vi "Logika case v13.vi"() -> ()   [LabVIEW 2014]
uses:
  Timer/Timer 2013/Control Timer.ctl
panel:
  in  "lokalna B3":bool
  out "Trenutno stanje":T1(ring)
  out "flag":dbl
  out "error out":errorcluster
  in  "error in (no error)":errorcluster
  in  "Stanja":T1(ring)
  in  "Flag":enum16{"1", "2", "3"}(ring)
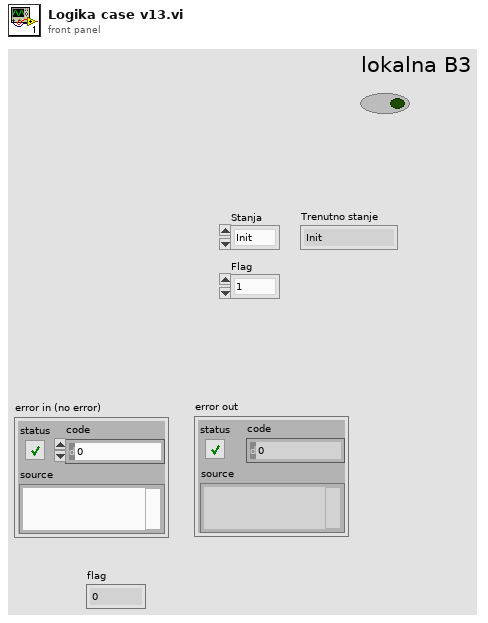
[diagram p1: front panel]
types:
  T1 = enum16{"Init", "Wait", "na1", "na2", "na3", "ispredLifta", "idiNaLift", "naLiftu", "uNivou1", "stigao1", "podizanje", "uNivou2", "stigao2", "uNivou3", "stigao3", "SHUTDOWN", "visak1", "visak2", "visak3"}
  T2 = typedef "Control Timer.ctl" = enum16{"Timecheck", "Reset"}
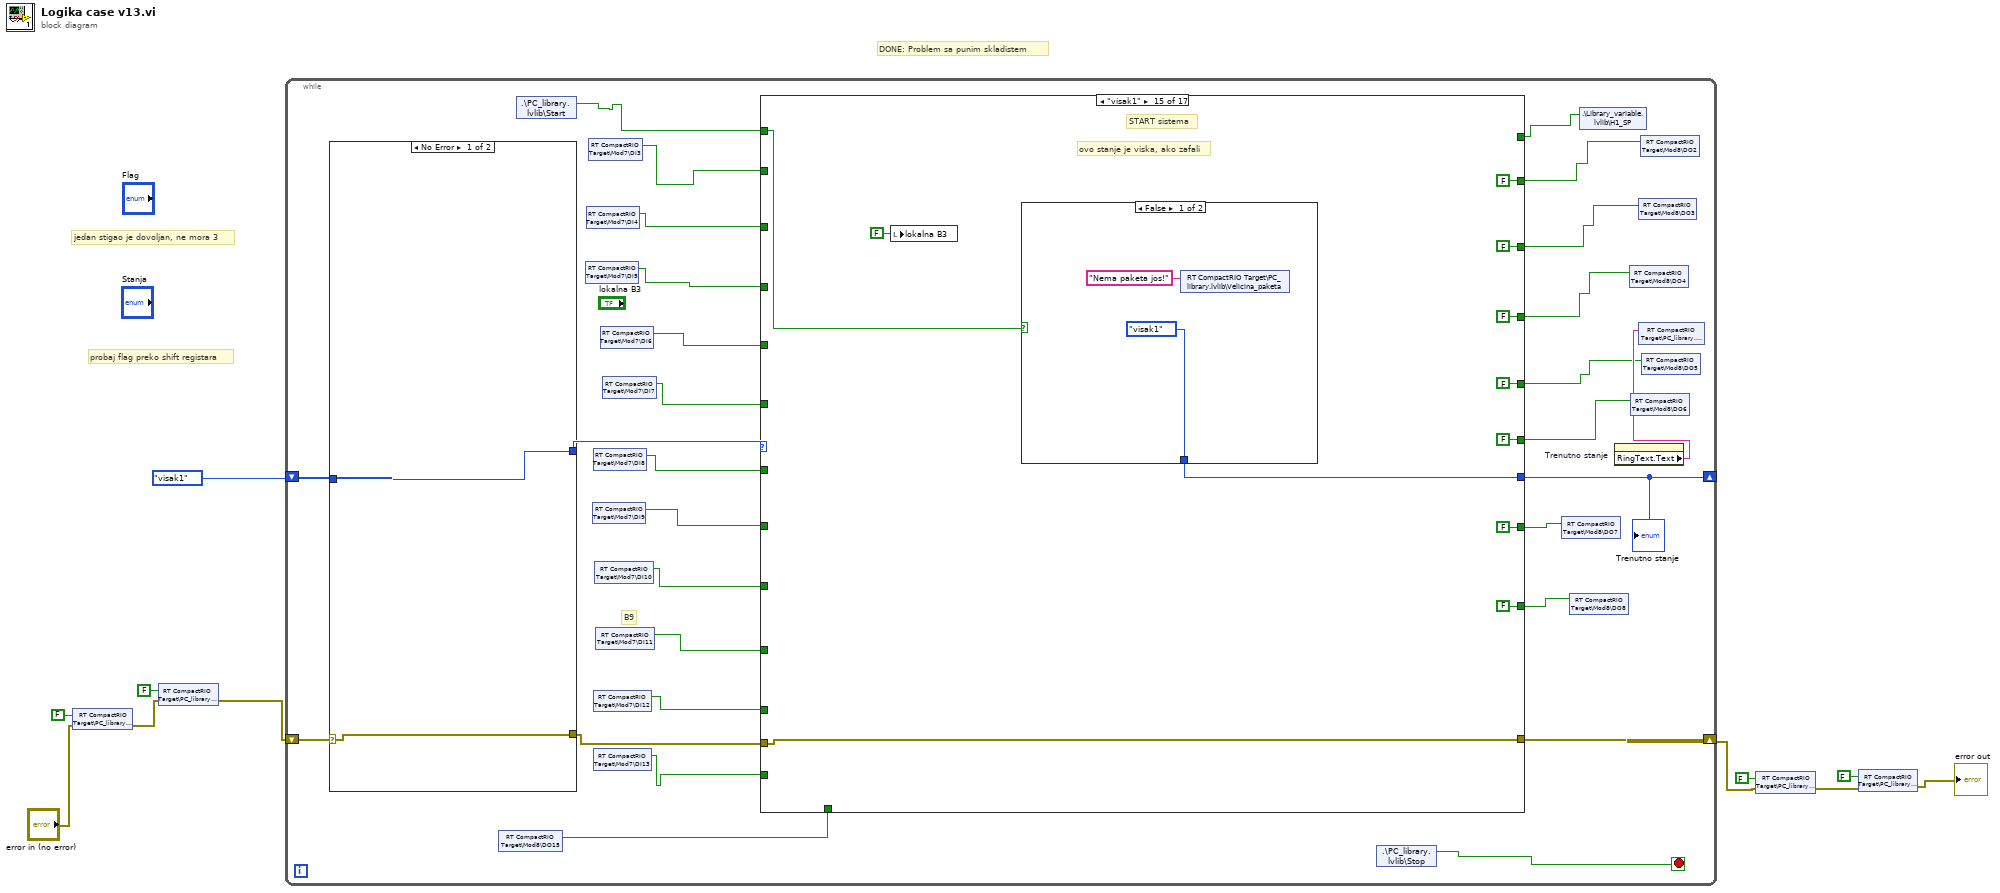
[diagram p0: block diagram]
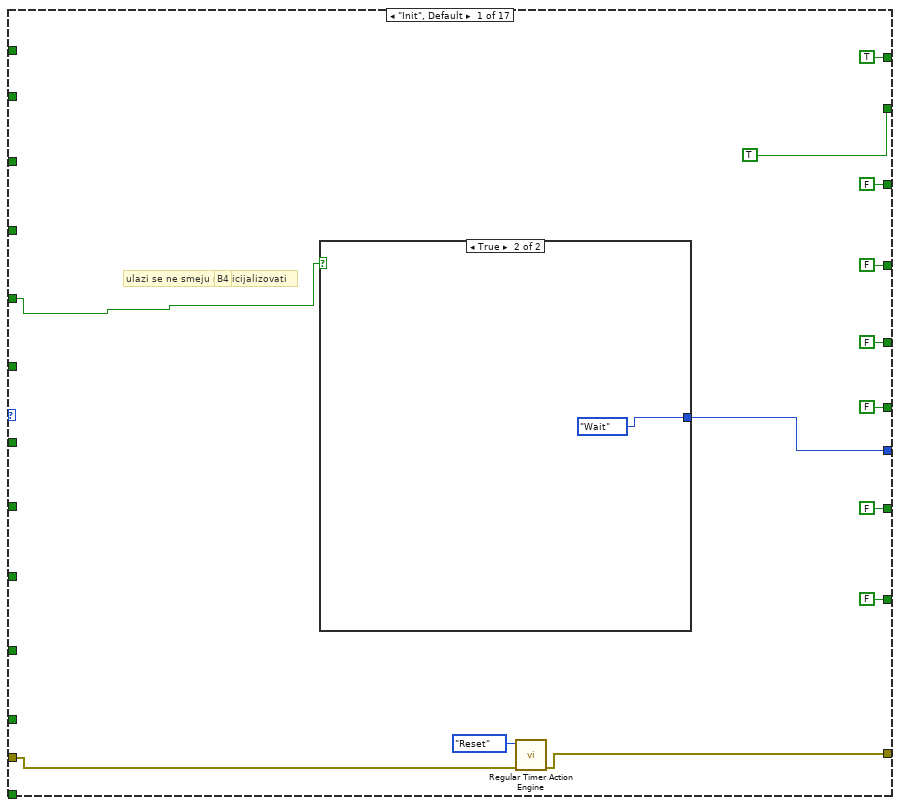
[diagram p2: hidden frame]
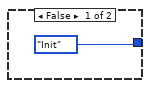
[diagram p3: hidden frame]
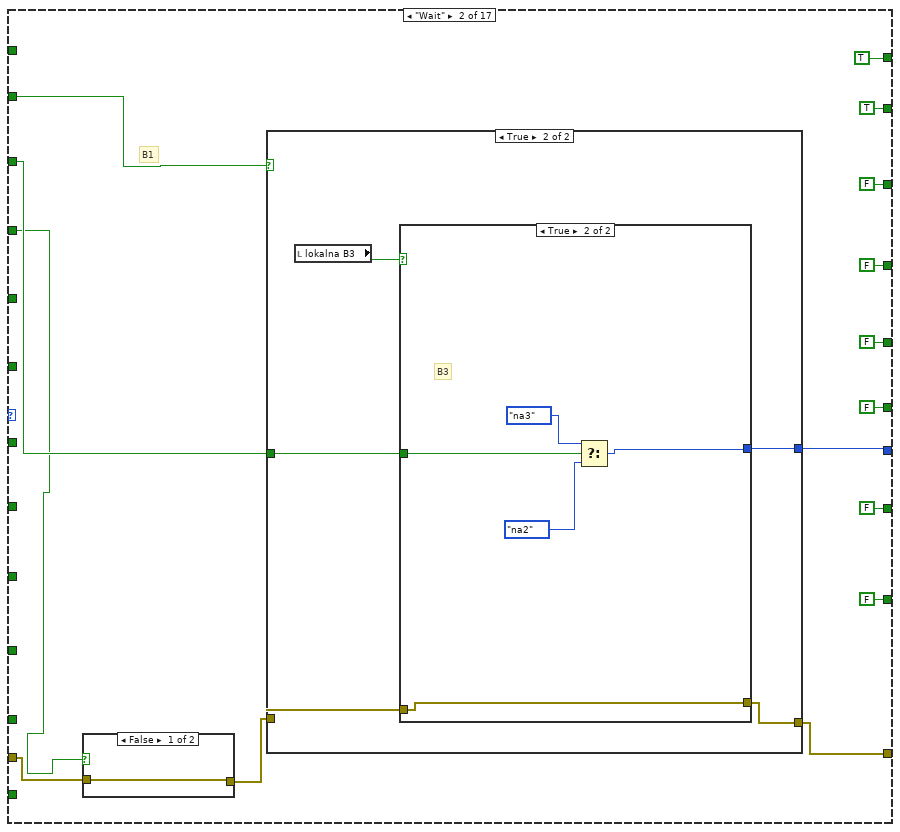
[diagram p4: hidden frame]
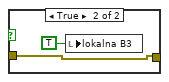
[diagram p5: hidden frame]
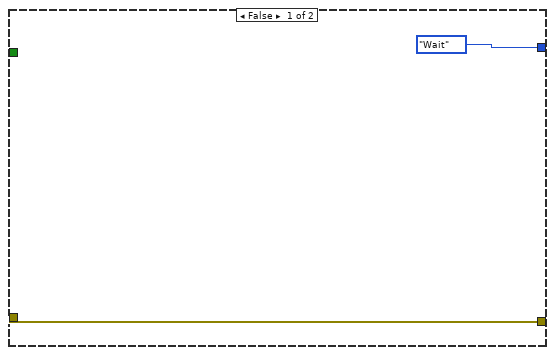
[diagram p6: hidden frame]
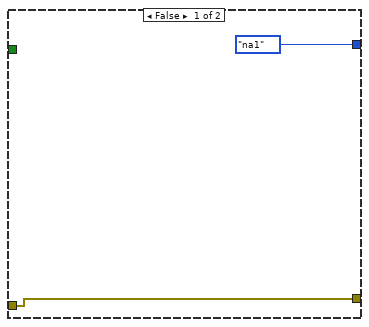
[diagram p7: hidden frame]
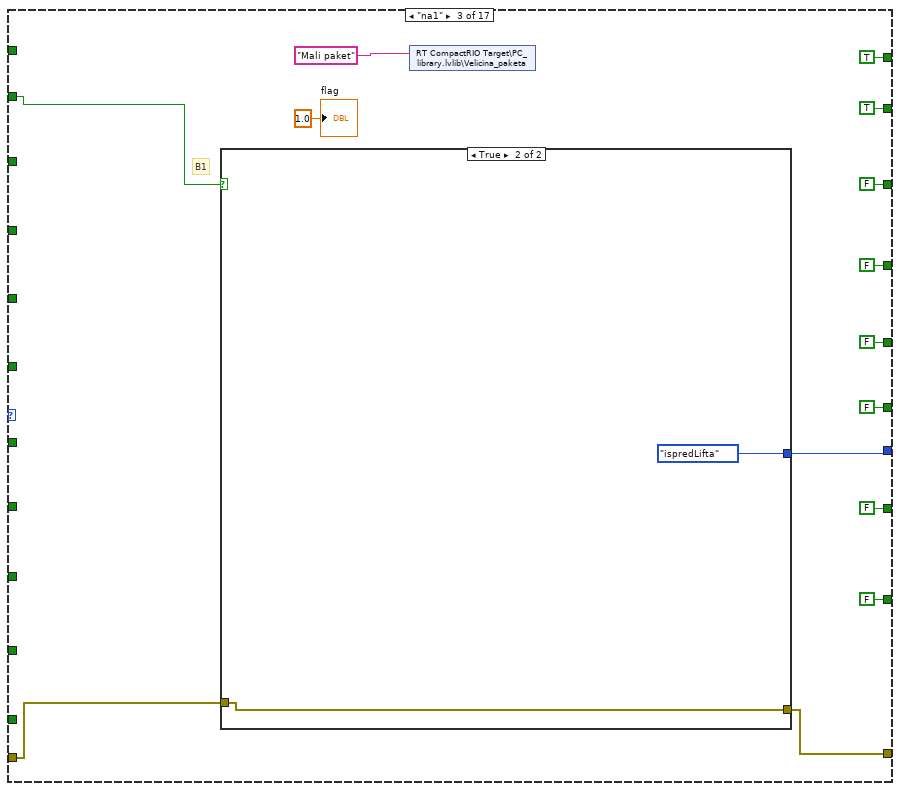
[diagram p8: hidden frame]
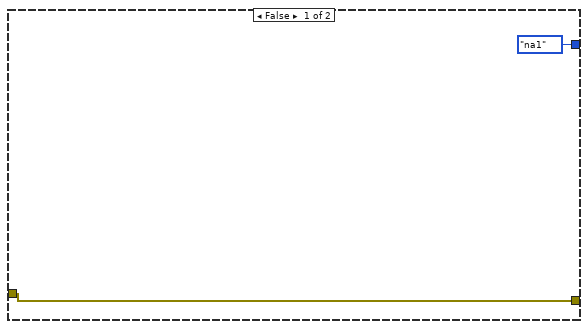
[diagram p9: hidden frame]
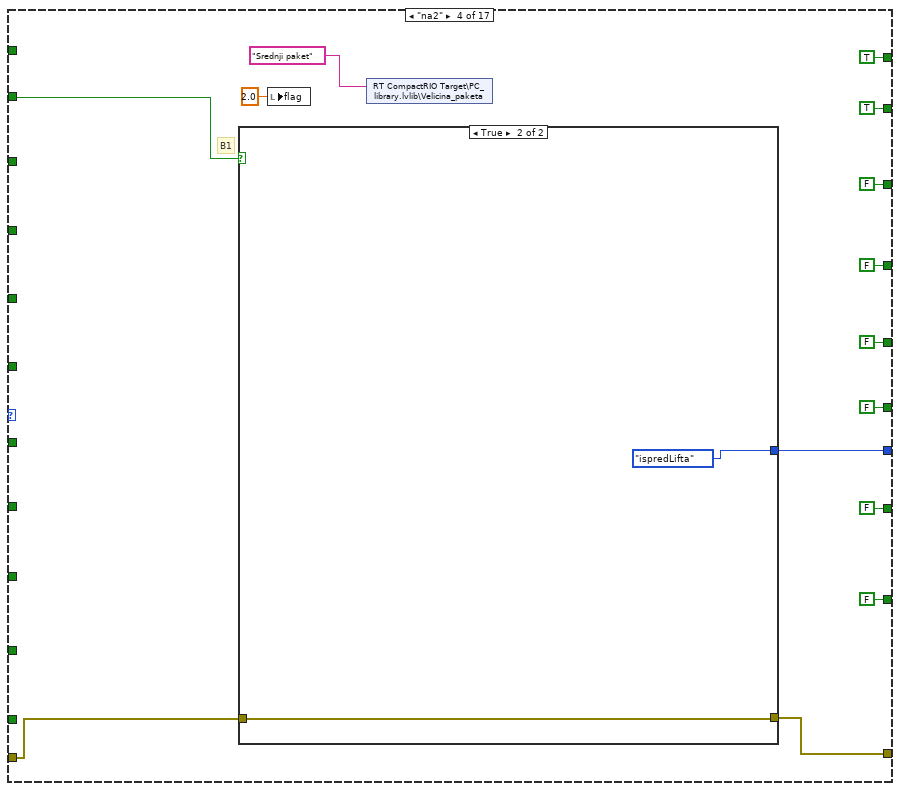
[diagram p10: hidden frame]
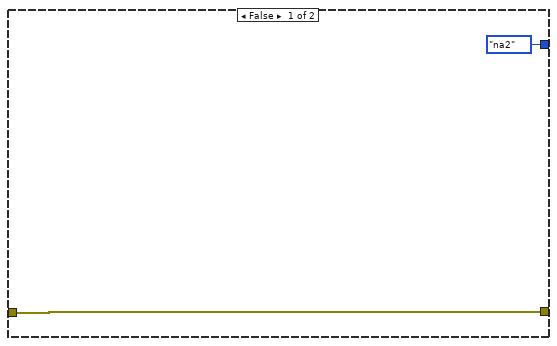
[diagram p11: hidden frame]
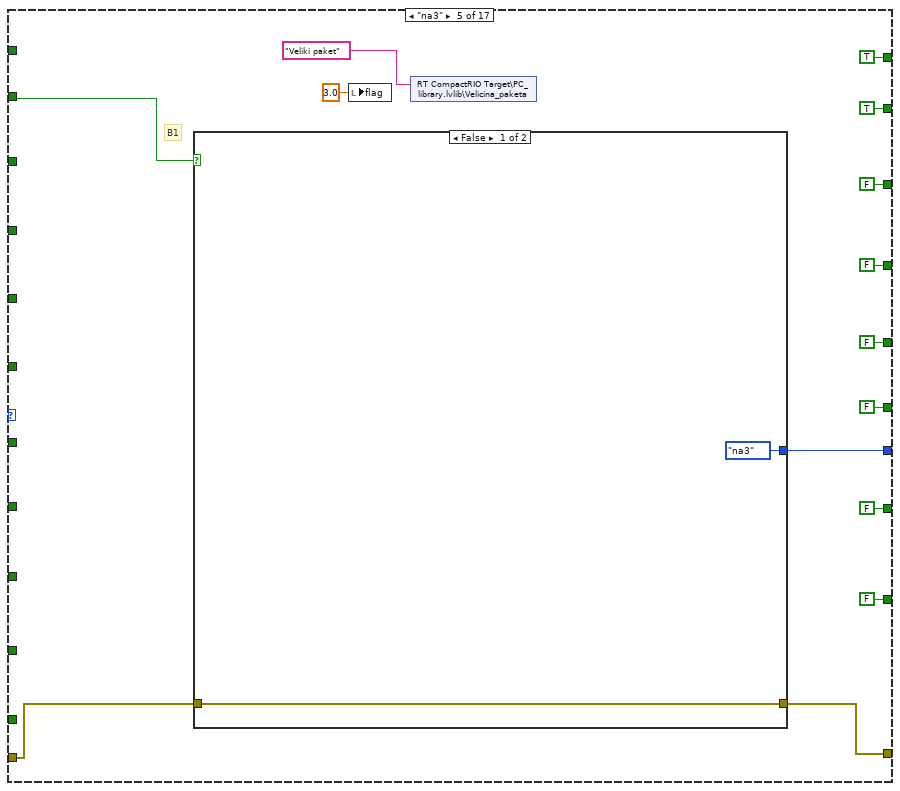
[diagram p12: hidden frame]
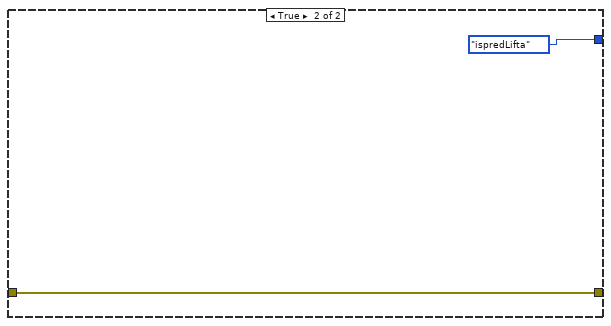
[diagram p13: hidden frame]
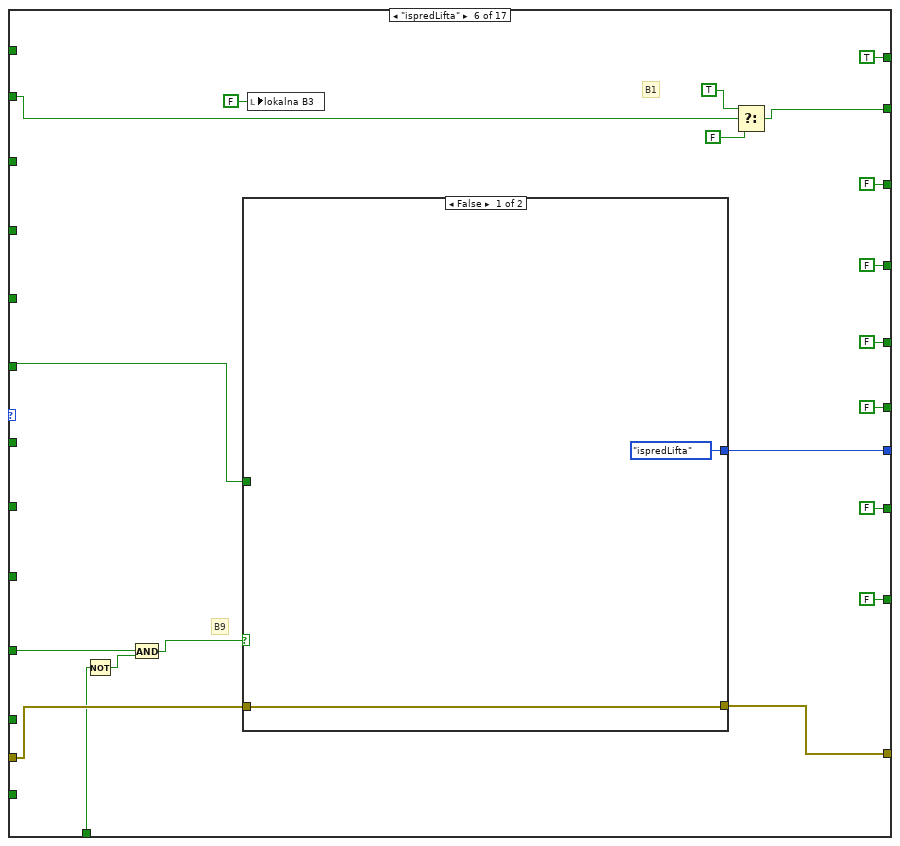
[diagram p14: hidden frame]
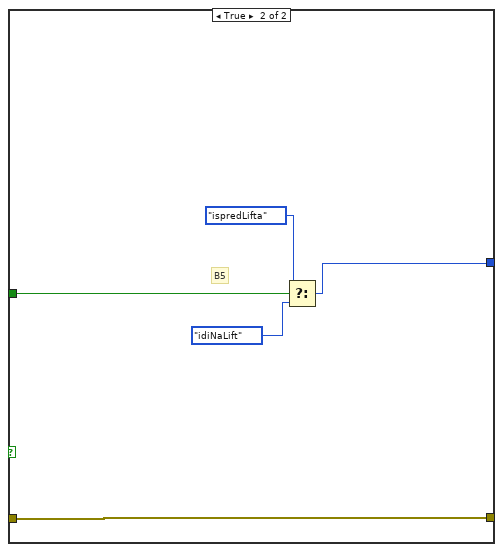
[diagram p15: hidden frame]
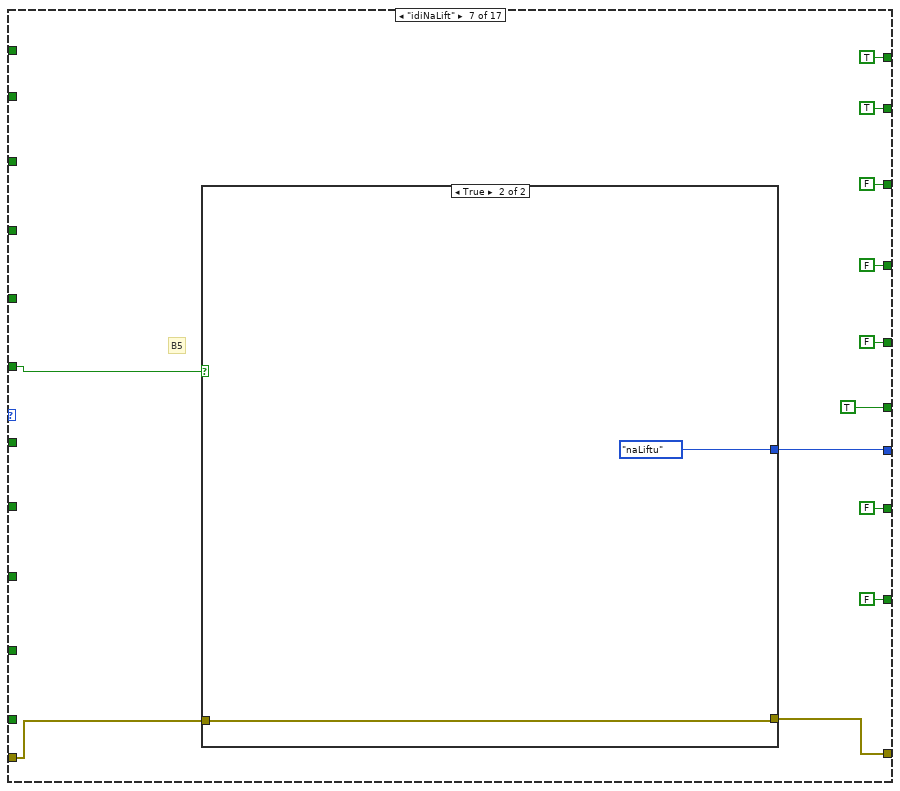
[diagram p16: hidden frame]
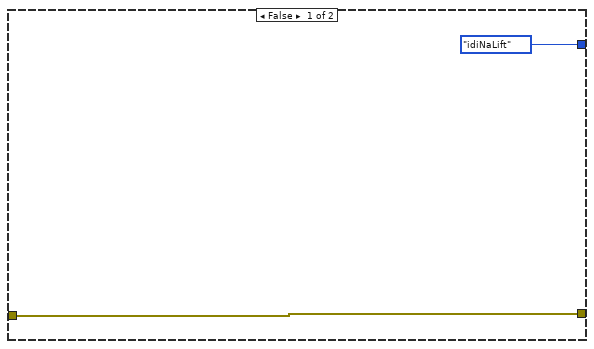
[diagram p17: hidden frame]
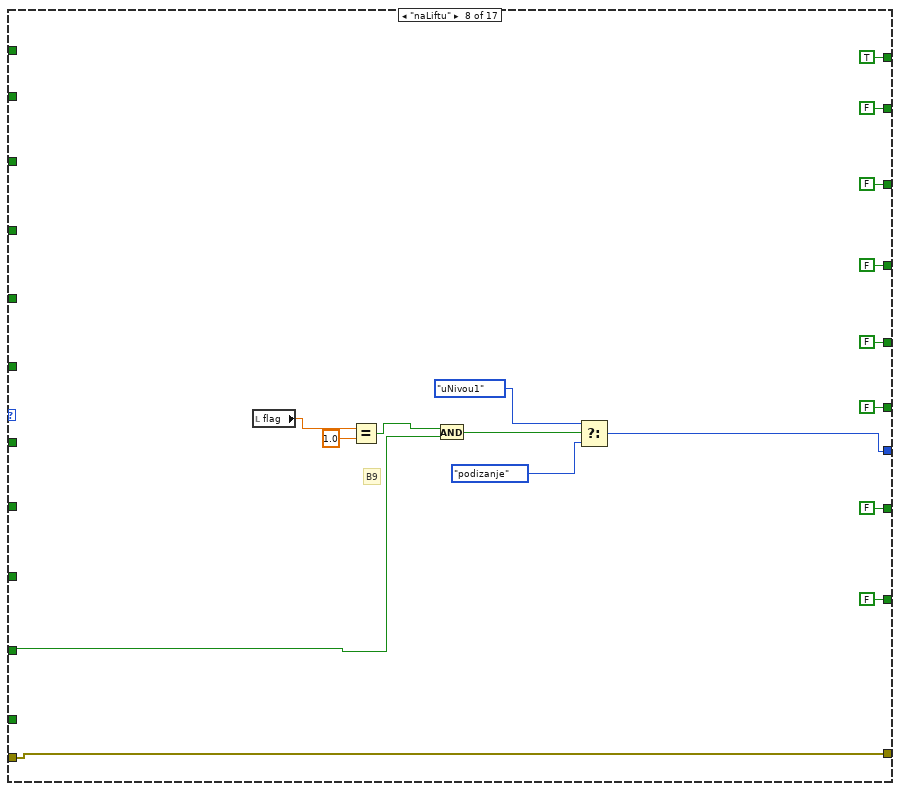
[diagram p18: hidden frame]
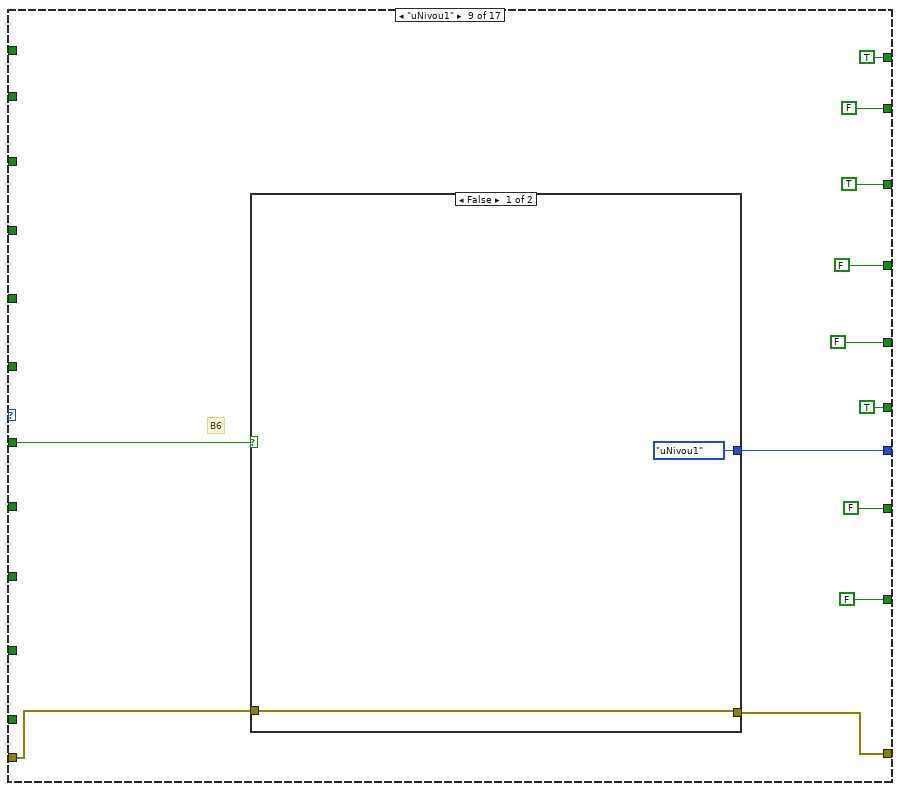
[diagram p19: hidden frame]
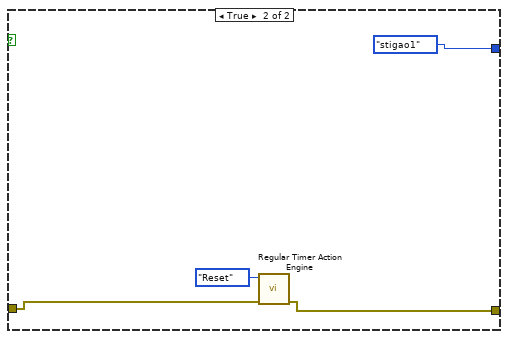
[diagram p20: hidden frame]
diagram:
  # "DONE: Problem sa punim skladistem"
  # "probaj flag preko shift registara"
  # "jedan stigao je dovoljan, ne mora 3"
  n1 = shared-variable "RT CompactRIO Target\\PC_library.lvlib\\Stop"(FALSE ("Stop"), error in="error in (no error)") -> (error out=w5:errorcluster)
  n2 = shared-variable "RT CompactRIO Target\\PC_library.lvlib\\Start"(FALSE ("Start"), error in=w5) -> (error out=w4:errorcluster)
  n3 = while {
    shift-right: [w36] -> w7
    shift-left: w4 -> [w40]
    shift-right: [w35] -> _
    shift-left: T1."visak1" ("Stanja") -> [w38]
    stop <- w33 stop-if-true
    # "B9"
    n4 = case shown="No Error" w40 {
      selector: w40 -> [w384 w385]
      tunnel: [w384 w385] -> w37
      tunnel: [w383 T1."SHUTDOWN" ("Stanja")] -> w39
      tunnel: w38 -> [w383 _]
      frame No Error {
      }
      frame Error {
      }
    }
    n5 = shared-variable "RT CompactRIO Target\\Mod8\\DO15"() -> (w12:bool)  [unwired: 1 in, 1 out]
    n6 = shared-variable ".\\PC_library.lvlib\\Start"() -> (w32:bool)  [unwired: 1 in, 1 out]
    n7 = shared-variable "RT CompactRIO Target\\Mod7\\DI5"() -> (w22:bool)  [unwired: 1 in, 1 out]
    n8 = shared-variable "RT CompactRIO Target\\Mod7\\DI4"() -> (w21:bool)  [unwired: 1 in, 1 out]
    n9 = shared-variable "RT CompactRIO Target\\Mod7\\DI3"() -> (w20:bool)  [unwired: 1 in, 1 out]
    n10 = shared-variable "RT CompactRIO Target\\Mod7\\DI9"() -> (w26:bool)  [unwired: 1 in, 1 out]
    n11 = shared-variable "RT CompactRIO Target\\Mod7\\DI8"() -> (w25:bool)  [unwired: 1 in, 1 out]
    n12 = shared-variable "RT CompactRIO Target\\Mod7\\DI12"() -> (w29:bool)  [unwired: 1 in, 1 out]
    n13 = shared-variable "RT CompactRIO Target\\Mod7\\DI13"() -> (w30:bool)  [unwired: 1 in, 1 out]
    n14 = shared-variable "RT CompactRIO Target\\Mod7\\DI10"() -> (w27:bool)  [unwired: 1 in, 1 out]
    n15 = shared-variable "RT CompactRIO Target\\Mod7\\DI11"() -> (w28:bool)  [unwired: 1 in, 1 out]
    n16 = shared-variable "RT CompactRIO Target\\Mod7\\DI6"() -> (w23:bool)  [unwired: 1 in, 1 out]
    n17 = shared-variable "RT CompactRIO Target\\Mod7\\DI7"() -> (w24:bool)  [unwired: 1 in, 1 out]
    n18 = case shown="\"visak1\"" w39 {
      selector: w39 -> [_ _ _ _ _ _ _ _ _ _ _ _ _ w343 _ w373 w382]
      tunnel: [TRUE TRUE TRUE TRUE TRUE w150 TRUE FALSE FALSE FALSE FALSE FALSE FALSE FALSE FALSE FALSE FALSE] -> w13
      tunnel: [w47 w69 w100 w118 w136 w161 w178 w194 w206 w243 w286 w311 w331 w343 w352 w373 w382] -> w35
      tunnel: w37 -> [w44 w56 w91 w109 w127 w153 w171 w193 w204 w230 w277 w306 w322 w340 w361 w372 w381]
      tunnel: [w45 w62 w92 w110 w128 w154 w172 w193 w205 w226 w278 w307 w323 w339 w361 w372 w381] -> w36
      tunnel: [FALSE FALSE FALSE FALSE FALSE FALSE TRUE FALSE TRUE FALSE FALSE TRUE TRUE FALSE FALSE FALSE FALSE] -> w17
      tunnel: [FALSE FALSE FALSE FALSE FALSE FALSE FALSE FALSE TRUE w233 FALSE FALSE FALSE FALSE FALSE FALSE FALSE] -> w14
      tunnel: [FALSE FALSE FALSE FALSE FALSE FALSE FALSE FALSE FALSE w232 FALSE TRUE FALSE FALSE FALSE FALSE FALSE] -> w15
      tunnel: [FALSE FALSE FALSE FALSE FALSE FALSE FALSE FALSE FALSE w231 FALSE FALSE TRUE FALSE FALSE FALSE FALSE] -> w16
      tunnel: [FALSE FALSE FALSE FALSE FALSE FALSE FALSE FALSE FALSE w222 FALSE FALSE FALSE FALSE FALSE FALSE FALSE] -> w18
      tunnel: [FALSE FALSE FALSE FALSE FALSE FALSE FALSE FALSE FALSE FALSE TRUE FALSE FALSE FALSE FALSE FALSE FALSE] -> w19
      tunnel: w20 -> [_ w60 w90 w108 w126 w148 _ _ _ _ _ _ _ _ _ _ _]
      tunnel: w21 -> [_ w58 _ _ _ _ _ _ _ _ _ _ _ _ _ _ _]
      tunnel: w22 -> [_ w57 _ _ _ _ _ _ _ _ _ _ _ _ _ _ _]
      tunnel: w23 -> [w42 _ _ _ _ _ _ _ _ _ _ _ _ _ _ _ _]
      tunnel: w24 -> [_ _ _ _ _ w149 w170 _ _ _ _ _ _ _ _ _ _]
      tunnel: w25 -> [_ _ _ _ _ _ _ _ w203 _ _ _ _ _ _ _ _]
      tunnel: w26 -> [_ _ _ _ _ _ _ _ _ _ _ w305 _ _ _ _ _]
      tunnel: w27 -> [_ _ _ _ _ _ _ _ _ _ _ _ w321 _ _ _ _]
      tunnel: w28 -> [_ _ _ _ _ w146 _ w186 _ w221 _ _ _ _ _ _ _]
      tunnel: w29 -> [_ _ _ _ _ _ _ _ _ _ w276 _ _ _ _ _ _]
      tunnel: w30 -> [_ _ _ _ _ _ _ _ _ _ w275 _ _ _ _ _ _]
      tunnel: w32 -> [_ _ _ _ _ _ _ _ _ _ _ _ _ _ w353 _ _]
      tunnel: [TRUE ("Start") TRUE TRUE ("Start") TRUE ("Start") TRUE ("Start") TRUE ("Start") TRUE ("Start") TRUE ("Start") TRUE ("Start") TRUE ("Start") TRUE ("Start") TRUE ("Start") TRUE ("Start") FALSE ("Start") _ _ _] -> w31
      tunnel: w12 -> [_ _ _ _ _ w144 _ _ _ _ _ _ _ _ _ _ _]
      frame "Init", Default {
        # "ulazi se ne smeju reinicijalizovati"
        # "B4"
        n19 = case shown="True" w42 {
          tunnel: [T1."Init" ("Stanja") T1."Wait" ("Stanja")] -> w47
          frame False {
          }
          frame True {
          }
        }
        n20 = call "Regular Timer Action Engine.vi"("Enum"=Control_Timer."Reset", "error in"=w44) -> ("error out"=w45:errorcluster)  [unwired: 7 in, 1 out]
      }
      frame "Wait" {
        # "B1"
        n21 = case shown="False" w57 {
          tunnel: [w71 w72] -> w59
          tunnel: w56 -> [w71 w72]
          frame False {
          }
          frame True {
            n22 = local write "lokalna B3"(TRUE ("lokalna B3")) -> ()
          }
        }
        n23 = case shown="True" w60 {
          tunnel: [T1."Wait" ("Stanja") w80] -> w69
          tunnel: w59 -> [w75 w79]
          tunnel: [w75 w78] -> w62
          tunnel: w58 -> [_ w76]
          frame False {
          }
          frame True {
            n24 = local read "lokalna B3"() -> (w77:bool)
            n25 = case shown="True" w77 {
              tunnel: [T1."na1" ("Stanja") w85] -> w80
              tunnel: w79 -> [w81 w84]
              tunnel: [w81 w84] -> w78
              tunnel: w76 -> [_ w83]
              frame False {
              }
              frame True {
                # "B3"
                n26 = Select(t=T1."na3" ("Stanja"), s=w83, f=T1."na2" ("Stanja")) -> (s? t:f=w85:T1)
              }
            }
          }
        }
      }
      frame "na1" {
        # "B1"
        n27 = case shown="True" w90 {
          tunnel: [T1."na1" ("Stanja") T1."ispredLifta" ("Stanja")] -> w100
          tunnel: [w102 w104] -> w92
          tunnel: w91 -> [w102 w104]
          frame False {
          }
          frame True {
          }
        }
        n28 = shared-variable "RT CompactRIO Target\\PC_library.lvlib\\Velicina_paketa"("Mali paket") -> ()  [unwired: 1 in, 1 out]
        "flag" <- 1.0 ("flag")
      }
      frame "na2" {
        # "B1"
        n29 = case shown="True" w108 {
          tunnel: [T1."na2" ("Stanja") T1."ispredLifta" ("Stanja")] -> w118
          tunnel: [w120 w122] -> w110
          tunnel: w109 -> [w120 w122]
          frame False {
          }
          frame True {
          }
        }
        n30 = local write "flag"(2.0 ("flag")) -> ()
        n31 = shared-variable "RT CompactRIO Target\\PC_library.lvlib\\Velicina_paketa"("Srednji paket") -> ()  [unwired: 1 in, 1 out]
      }
      frame "na3" {
        # "B1"
        n32 = case shown="False" w126 {
          tunnel: [T1."na3" ("Stanja") T1."ispredLifta" ("Stanja")] -> w136
          tunnel: [w138 w140] -> w128
          tunnel: w127 -> [w138 w140]
          frame False {
          }
          frame True {
          }
        }
        n33 = local write "flag"(3.0 ("flag")) -> ()
        n34 = shared-variable "RT CompactRIO Target\\PC_library.lvlib\\Velicina_paketa"("Veliki paket" ("Velicina_Paketa")) -> ()  [unwired: 1 in, 1 out]
      }
      frame "ispredLifta" {
        # "B1"
        # "B9"
        n35 = Not(x=w144) -> (.not. x?=w145:bool)
        n36 = And(x=w146, y=w145) -> (x .and. y?=w143:bool)
        n37 = case shown="False" w143 {
          tunnel: [T1."ispredLifta" ("Stanja") w168] -> w161
          tunnel: [w162 w165] -> w154
          tunnel: w153 -> [w162 w165]
          tunnel: w149 -> [_ w164]
          frame False {
          }
          frame True {
            # "B5"
            n38 = Select(t=T1."ispredLifta" ("Stanja"), s=w164, f=T1."idiNaLift" ("Stanja")) -> (s? t:f=w168:T1)
          }
        }
        n39 = local write "lokalna B3"(FALSE ("lokalna B3")) -> ()
        n40 = Select(t=TRUE, s=w148, f=FALSE) -> (s? t:f=w150:bool)
      }
      frame "idiNaLift" {
        # "B5"
        n41 = case shown="True" w170 {
          tunnel: [T1."idiNaLift" ("Stanja") T1."naLiftu" ("Stanja")] -> w178
          tunnel: [w181 w183] -> w172
          tunnel: w171 -> [w181 w183]
          frame False {
          }
          frame True {
          }
        }
      }
      frame "naLiftu" {
        # "B9"
        n42 = local read "flag"() -> (w200:dbl)
        n43 = Equal?(x=w200, y=1.0) -> (x = y?=w198:bool)
        n44 = And(x=w198, y=w186) -> (x .and. y?=w197:bool)
        n45 = Select(t=T1."uNivou1" ("Stanja"), s=w197, f=T1."podizanje" ("Stanja")) -> (s? t:f=w194:T1)
      }
      frame "uNivou1" {
        # "B6"
        n46 = case shown="False" w203 {
          tunnel: [T1."uNivou1" ("Stanja") T1."stigao1" ("Stanja")] -> w206
          tunnel: [w214 w216] -> w205
          tunnel: w204 -> [w214 w217]
          frame False {
          }
          frame True {
            n47 = call "Regular Timer Action Engine.vi"("Enum"=Control_Timer."Reset", "error in"=w217) -> ("error out"=w216:errorcluster)  [unwired: 7 in, 1 out]
          }
        }
      }
      frame "stigao1" {
        # "B9"
        # "K2, K3 i K4 ce vrv\nbiti upravljani preko\nDone iz tajmera"
        # "ako nije na prvom\nspratu, spustaj"
        n48 = call "Regular Timer Action Engine.vi"("Enum"=Control_Timer."Timecheck", "Time Target"=20.0, "error in"=w230) -> ("Status"=w236:cluster{"Running":bool, "Done":bool}, "error out"=w229:errorcluster)  [unwired: 6 in]
        n49 = Unbundle(w236) -> ("Running"=w234:bool, "Done"=w225:bool)
        n50 = case shown="True" w225 {
          tunnel: [T1."stigao1" ("Stanja") w249] -> w243
          tunnel: w221 -> [_ w248]
          tunnel: w230 -> [w245 w247]
          tunnel: [w245 w246] -> w227
          frame False {
          }
          frame True {
            n51 = case shown="True" w248 {
              tunnel: [T1."stigao1" ("Stanja") T1."Wait" ("Stanja")] -> w249
              tunnel: [w250 w253] -> w246
              tunnel: w247 -> [w250 w254]
              frame False {
              }
              frame True {
                n52 = call "Regular Timer Action Engine.vi"("Enum"=Control_Timer."Reset", "error in"=w254) -> ("error out"=w253:errorcluster)  [unwired: 7 in, 1 out]
              }
            }
          }
        }
        n53 = case shown="True" w234 {
          tunnel: [FALSE w263] -> w233
          tunnel: [FALSE w262] -> w232
          tunnel: [FALSE w261] -> w231
          tunnel: w229 -> [w256 w260]
          tunnel: [w256 w260] -> w228
          frame False {
          }
          frame True {
            n54 = local read "flag"() -> (w264:dbl)
            n55 = case shown="1, Default" w264 {
              tunnel: [TRUE FALSE FALSE] -> w263
              tunnel: [FALSE TRUE FALSE] -> w262
              tunnel: [FALSE FALSE TRUE] -> w261
              frame 1, Default {
              }
              frame 2 {
              }
              frame 3 {
              }
            }
          }
        }
        n56 = Not(x=w221) -> (.not. x?=w220:bool)
        n57 = local read "flag"() -> (w238:dbl)
        n58 = Merge Errors(w228, w227) -> (w226:errorcluster)
        n59 = Not Equal?(x=w238, y=1.0) -> (x != y?=w223:bool)
        n60 = And(x=w223, y=w220) -> (x .and. y?=w222:bool)
      }
      frame "podizanje" {
        # "B10"
        n61 = local read "flag"() -> (w290:dbl)
        n62 = Equal?(x=w290, y=2.0) -> (x = y?=w288:bool)
        n63 = And(x=w288, y=w276) -> (x .and. y?=w287:bool)
        n64 = case shown="False" w287 {
          tunnel: [w293 T1."uNivou2" ("Stanja")] -> w286
          tunnel: [w292 w300] -> w278
          tunnel: w277 -> [w292 w300]
          tunnel: w275 -> [w291 _]
          frame False {
            # "B11"
            n65 = local read "flag"() -> (w298:dbl)
            n66 = Equal?(x=w298, y=3.0) -> (x = y?=w299:bool)
            n67 = And(x=w299, y=w291) -> (x .and. y?=w296:bool)
            n68 = Select(t=T1."uNivou3" ("Stanja"), s=w296, f=T1."podizanje" ("Stanja")) -> (s? t:f=w293:T1)
          }
          frame True {
          }
        }
      }
      frame "uNivou2" {
        # "B7"
        n69 = case shown="True" w305 {
          tunnel: [T1."uNivou2" ("Stanja") T1."stigao1" ("Stanja")] -> w311
          tunnel: [w315 w316] -> w307
          tunnel: w306 -> [w315 w317]
          frame False {
          }
          frame True {
            n70 = call "Regular Timer Action Engine.vi"("Enum"=Control_Timer."Reset", "error in"=w317) -> ("error out"=w316:errorcluster)  [unwired: 7 in, 1 out]
          }
        }
      }
      frame "uNivou3" {
        # "B8"
        n71 = case shown="True" w321 {
          tunnel: [T1."uNivou3" ("Stanja") T1."stigao1" ("Stanja")] -> w331
          tunnel: [w332 w334] -> w323
          tunnel: w322 -> [w332 w335]
          frame False {
          }
          frame True {
            n72 = call "Regular Timer Action Engine.vi"("Enum"=Control_Timer."Reset", "error in"=w335) -> ("error out"=w334:errorcluster)  [unwired: 7 in, 1 out]
          }
        }
      }
      frame "SHUTDOWN" {
        n73 = shared-variable "RT CompactRIO Target\\PC_library.lvlib\\Start"(FALSE ("Start"), error in=w340) -> (error out=w339:errorcluster)
        n74 = shared-variable "RT CompactRIO Target\\PC_library.lvlib\\Velicina_paketa"("Nema paketa jos!" ("Velicina_paketa")) -> ()  [unwired: 1 in, 1 out]
      }
      frame "visak1" {
        # "START sistema"
        # "ovo stanje je viska, ako zafali"
        n75 = local write "lokalna B3"(FALSE ("lokalna B3")) -> ()
        n76 = case shown="False" w353 {
          tunnel: [T1."visak1" ("Stanja") T1."Init" ("Stanja")] -> w352
          frame False {
            n77 = shared-variable "RT CompactRIO Target\\PC_library.lvlib\\Velicina_paketa"("Nema paketa jos!" ("Velicina_paketa")) -> ()  [unwired: 1 in, 1 out]
          }
          frame True {
          }
        }
      }
      frame "visak2" {
        # "ovo stanje je viska, ako zafali"
      }
      frame "visak3" {
        # "ovo stanje je viska, ako zafali"
      }
    }
    "Trenutno stanje" <- w35
    n78 = shared-variable ".\\PC_library.lvlib\\Stop"() -> (w33:bool)  [unwired: 1 in, 1 out]
    n79 = shared-variable "RT CompactRIO Target\\Mod8\\DO7"(w18) -> ()  [unwired: 1 in, 1 out]
    n80 = shared-variable "RT CompactRIO Target\\Mod8\\DO8"(w19) -> ()  [unwired: 1 in, 1 out]
    n81 = shared-variable ".\\Library_variable.lvlib\\H1_SP"(w31) -> ()  [unwired: 1 in, 1 out]
    n82 = property on="Trenutno stanje" class="Enum (strict)"() -> ("RingText.Text"=w34:string)  [unwired: 2 in, 2 out]
    n83 = shared-variable "RT CompactRIO Target\\Mod8\\DO4"(w15) -> ()  [unwired: 1 in, 1 out]
    n84 = shared-variable "RT CompactRIO Target\\Mod8\\DO6"(w17) -> ()  [unwired: 1 in, 1 out]
    n85 = shared-variable "RT CompactRIO Target\\Mod8\\DO3"(w14) -> ()  [unwired: 1 in, 1 out]
    n86 = shared-variable "RT CompactRIO Target\\PC_library.lvlib\\Stanje"(w34) -> ()  [unwired: 1 in, 1 out]
    n87 = shared-variable "RT CompactRIO Target\\Mod8\\DO2"(w13) -> ()  [unwired: 1 in, 1 out]
    n88 = shared-variable "RT CompactRIO Target\\Mod8\\DO5"(w16) -> ()  [unwired: 1 in, 1 out]
  }
  n89 = shared-variable "RT CompactRIO Target\\PC_library.lvlib\\Stop"(FALSE ("Stop"), error in=w7) -> (error out=w3:errorcluster)
  n90 = shared-variable "RT CompactRIO Target\\PC_library.lvlib\\Start"(FALSE ("Start"), error in=w3) -> (error out=→"error out":errorcluster)
